vi "locate mapping type array by action channel.vi"(7 "owner ID":string, 8 "error in":errorcluster, 10 "action channel":refnum<class "TBM channel.lvclass">, 11 "engine configuration in":refnum<class "base TBM sequencer configuration.lvclass">) -> (0 "error out":errorcluster, 1 "Mapping":T1, 2 "action channel out":refnum<class "TBM channel.lvclass">, 3 "engine configuration out":refnum<class "base TBM sequencer configuration.lvclass">)   [LabVIEW 2014, in "base TBM sequencer configuration.lvclass"]
uses:
  base TBM sequencer configuration.lvclass
  <vilib>/NI/Tag Bus Module Framework/channel/TBM channel.lvclass
  <vilib>/NI/Configuration Framework/NISE_CEF_TreeControl.lvlib
  <vilib>/NI/Tag Bus/tag/Data Type.ctl
  <vilib>/NI/Tag Bus/tag/tag descriptor.lvclass
  <vilib>/NI/Tag Bus/table/mapping.ctl
  <vilib>/NI/Tag Bus/table/data table.lvlib
  <vilib>/NI/Tag Bus/table/mapping specification.ctl
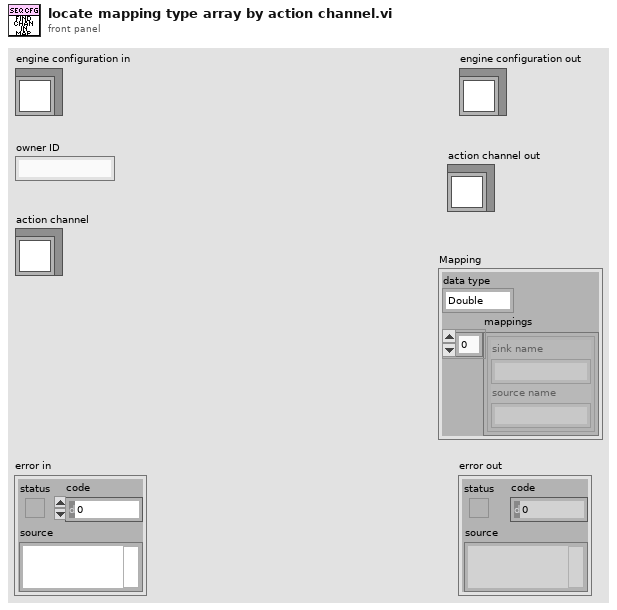
[diagram p1: front panel]
types:
  T1 = typedef "tag bus.lvlib/data table.lvlib/mapping specification.ctl" = cluster{"data type":T2, "mappings":T3[]}
  T2 = typedef "tag bus.lvlib/tag descriptor.lvclass/Data Type.ctl" = enum16{"Double", "Single", "I64", "I32", "I16", "I8", "U64", "U32", "U16", "U8", "Boolean", "String", "Array of Double", "Array of Single", "Array of I64", "Array of I32", "Array of I16", "Array of I8", "Array of U64", "Array of U32", "Array of U16", "Array of U8", "Array of Boolean", "Array of String"}
  T3 = typedef "tag bus.lvlib/data table.lvlib/mapping.ctl" = cluster{"sink name":string, "source name":string}
  T4 = typedef "base TBM sequencer configuration.lvclass/Module Mappings.ctl" = cluster{"Owning ID":string, "Input Mappings":T1[], "Process Parameter Mappings":T1[], "Process Results Mappings":T1[], "Output Mappings":T1[]}
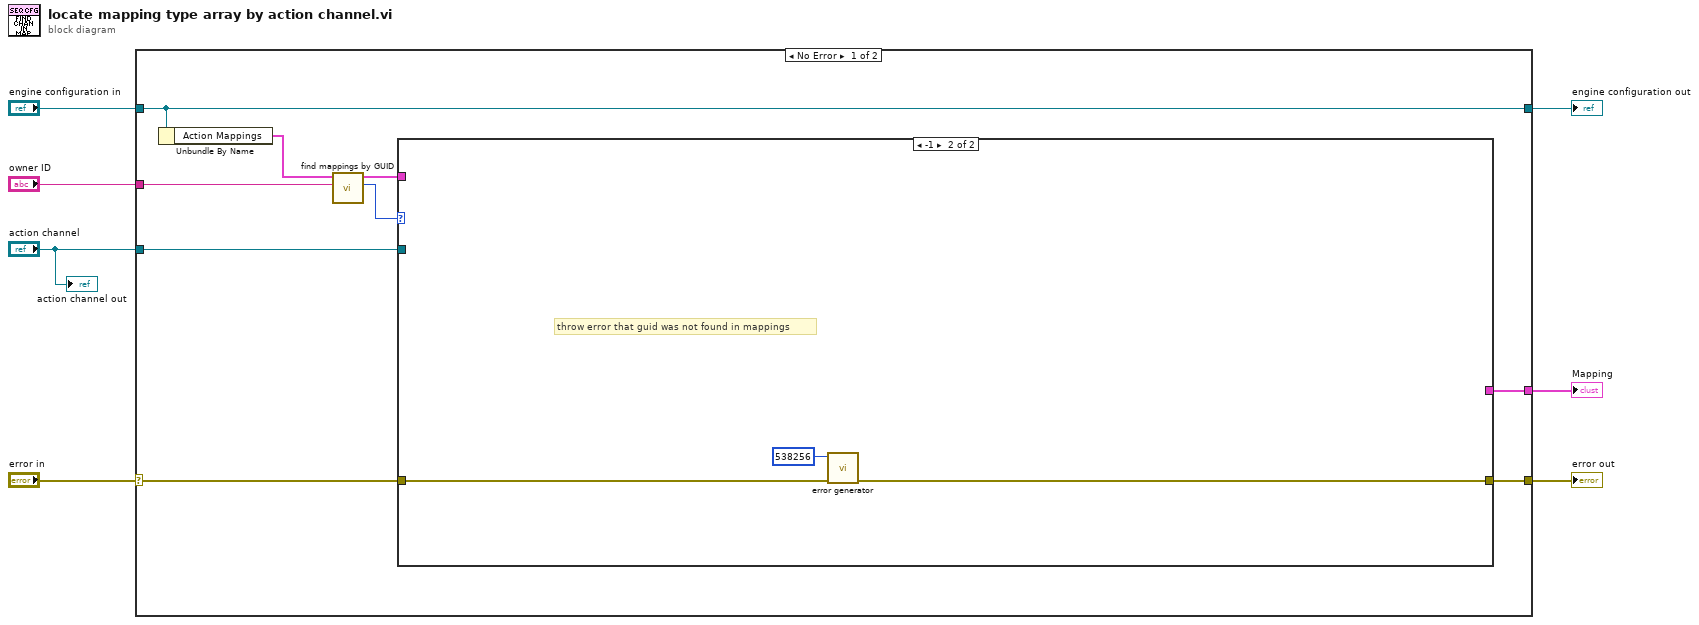
[diagram p0: block diagram]
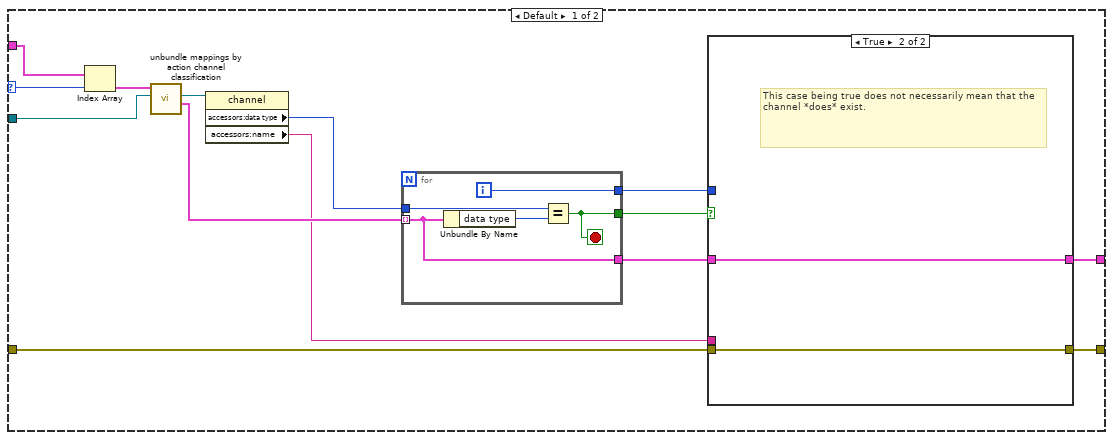
[diagram p2: hidden frame]
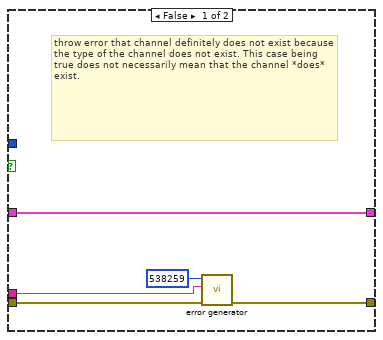
[diagram p3: hidden frame]
diagram:
  n1 = case shown="No Error" "error in" {
    selector: "error in" -> [w13 w47]
    tunnel: [w12 w47] -> w6
    tunnel: [w16 w46] -> w4
    tunnel: "engine configuration in" -> [w16 w46]
    tunnel: "owner ID" -> [w9 _]
    tunnel: "action channel" -> [w15 _]
    tunnel: [w14 _] -> w2
    frame No Error {
      n2 = Unbundle By Name(w16) -> ("Action Mappings"=w10:T4[])
      n3 = call "find mappings by GUID.vi"("owner ID"=w9, "action Mappings"=w10) -> ("index"=w8:i32, "action Mappings out"=w11:T4[])  [unwired: 8 in]
      n4 = case shown="-1" w8 {
        selector: w8 -> [w29 _]
        tunnel: w11 -> [w30 _]
        tunnel: w15 -> [w27 _]
        tunnel: [w20 _] -> w14
        tunnel: w13 -> [w19 w44]
        tunnel: [w18 w43] -> w12
        frame Default {
          n5 = Index Array(array=w30, index=w29) -> (element=w28:T4)
          n6 = call "unbundle mappings by action channel classification.vi"("channel"=w27, "Mappings"=w28) -> ("Mappings For One Method"=w24:T1[], "channel out"=w26:refnum<class "TBM channel.lvclass">)  [unwired: 7 in, 1 out]
          n7 = property class="channel"(reference=w26) -> ("accessors:data type"=w25:T2, "accessors:name"=w17:string)  [unwired: 1 in, 2 out]
          n8 = for {
            tunnel: w24 -> [w38] mode=indexing
            tunnel: w25 -> [w41]
            tunnel: [w40] -> w23
            tunnel: [w39] -> w22
            tunnel: [w38] -> w21
            i -> [w39]
            stop <- w40 stop-if-true
            n9 = Unbundle By Name(w38) -> ("data type"=w42:T2)
            n10 = Equal?(x=w41, y=w42) -> (x = y?=w40:bool)
          }
          n11 = case shown="True" w23 {
            tunnel: w22 -> [_ _]
            tunnel: w21 -> [w35 w36]
            tunnel: [w35 w36] -> w20
            tunnel: w19 -> [w33 w37]
            tunnel: [w32 w37] -> w18
            tunnel: w17 -> [w31 _]
            frame False {
              # "throw error that channel definitely does not exist because the type of the channel does not exist. This case being true does not necessarily mean that the channel *does* exist."
              n12 = call <vilib>:"error generator.vi"("error in"=w33, "append error message"=w31, "error code (0)"=538259) -> ("error out"=w32:errorcluster)  [unwired: 6 in]
            }
            frame True {
              # "This case being true does not necessarily mean that the channel *does* exist."
            }
          }
        }
        frame -1 {
          # "throw error that guid was not found in mappings"
          n13 = call <vilib>:"error generator.vi"("error in"=w44, "error code (0)"=538256) -> ("error out"=w43:errorcluster)  [unwired: 7 in]
        }
      }
    }
    frame Error {
    }
  }
  "error out" <- w6
  "engine configuration out" <- w4
  "Mapping" <- w2
  "action channel out" <- "action channel"
